vi "Read Optional Plane Type.vi"(9 "XYGraph in":refnum<class "XYGraph.lvclass">) -> (3 "XYGraph out":refnum<class "XYGraph.lvclass">, 4 "Optional Plane Type":T1(ring))   [LabVIEW 2014, in "Raspberry Pi Compatible Compiler for LabVIEW.lvlib" / "XYGraph.lvclass"]
uses:
  XYGraph.lvclass
  XYGraph.lvclass/XYGraph.ctl
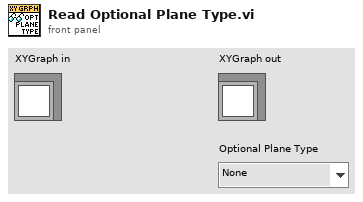
[diagram p1: front panel]
types:
  T1 = enum16{"None", "Nyquist", "Nichols", "S Plane", "Z Plane"}
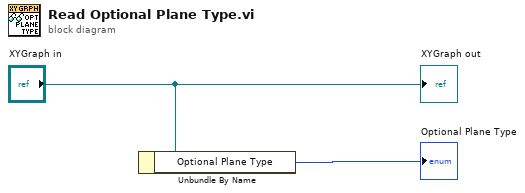
[diagram p0: block diagram]
diagram:
  n1 = Unbundle By Name("XYGraph in") -> ("Optional Plane Type"=→"Optional Plane Type":T1)
  "XYGraph out" <- "XYGraph in"
